vi "RQST Lookup Table Initialize.vi"(8 "error in (no error)":errorcluster) -> (0 "error out":errorcluster {"code" min=0 max=0}, 3 "reference out":T1)   [LabVIEW 2013, in "J1939 Addon Engine.lvlib"]
uses:
  Engine/J1939 Addon Engine.lvlib
  Types/RQST Lookup Table Reference.ctl
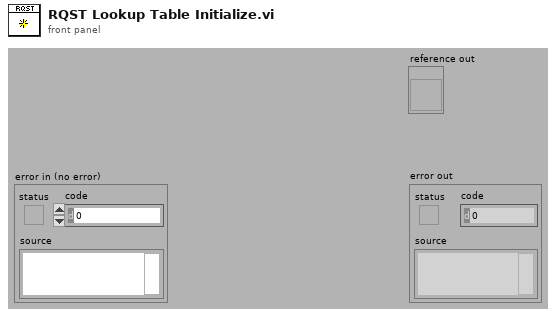
[diagram p1: front panel]
types:
  T1 = typedef "J1939 Addon Engine.lvlib/RQST Lookup Table Reference.ctl" = refnum<vi>
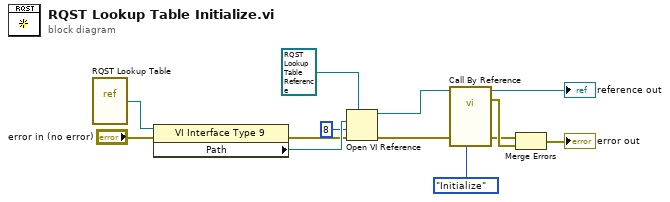
[diagram p0: block diagram]
diagram:
  n1 = vi-ref "RQST Lookup Table.vi"() -> (w13:refnum<vi>)
  n2 = property class="VI Interface Type 9"(reference=w13, error in="error in (no error)") -> (error out=w10:errorcluster, "Path"=w12:path)  [unwired: 1 out]
  n3 = Open VI Reference(type specifier VI Refnum (for type only)=T1 refnum ("reference out"), vi path=w12, options=8, error in (no error)=w10) -> (vi reference=w3:T1, error out=w6:errorcluster)  [unwired: 2 in]
  n4 = call-by-ref "?"(reference=w3, "Action"=enum16{"Initialize", "Add", "Get", "Remove"}."Initialize", "error in (no error)"=w6) -> (reference out=→"reference out":T1, error out=w9:errorcluster, 0:"error out"=w5:errorcluster)  [unwired: 8 in, 2 out]
  n5 = Merge Errors(w5, w9) -> (→"error out":errorcluster)
